vi "DAQmx Read (Raw 1D U16).vi"(0 "task/channels in":refnum<k21>, 7 "number of samples per channel":i32=-1, 9 "timeout":dbl=10.0 format="%0.2f", 11 "error in":errorcluster) -> (4 "task out":refnum<k21>, 6 "data":u16[](array[numeric]), 15 "error out":errorcluster)   [LabVIEW 2017]
doc: "Reads one or more raw, 16-bit unsigned integer samples from a task. Use this instance with devices that use 16-bit unsigned integers as the internal representation of a sample."
uses:
  nilvaiu.dll
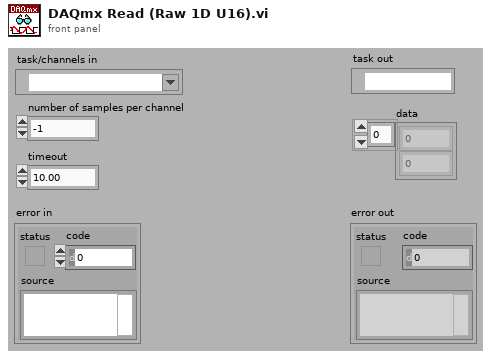
[diagram p1: front panel]
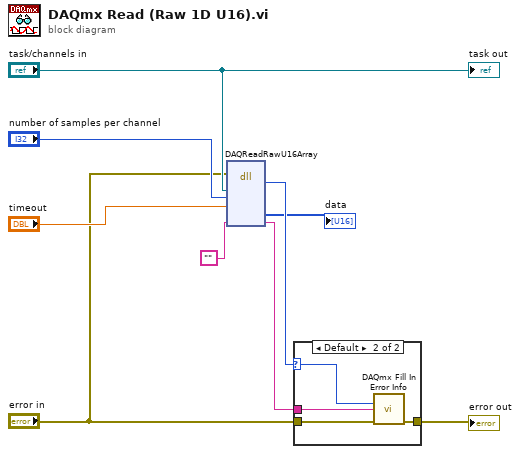
[diagram p0: block diagram]
diagram:
  n1 = dll-call lib="nilvaiu.*" fn="DAQReadRawU16Array"(error in="error in", "taskID"="task/channels in", "samplesPerChannel"="number of samples per channel", "timeout"="timeout", "extendedErrorInfo"="") -> ("return type"=w7:i32, "data"=→"data":u16[], "extendedErrorInfo"=w3:string)  [unwired: 5 in, 3 out]
  n2 = case shown="Default" w7 {
    selector: w7 -> [_ w12]
    tunnel: "error in" -> [w10 w14]
    tunnel: [w10 w13] -> w9
    tunnel: w3 -> [_ w11]
    frame 0 {
    }
    frame Default {
      n3 = call "DAQmx Fill In Error Info.vi"("status code"=w12, "extended error info"=w11, "error in"=w14) -> ("error out"=w13:errorcluster)  [unwired: 1 in, 11 out]
    }
  }
  "error out" <- w9
  "task out" <- "task/channels in"
